vi "fillWithZeros.vi"(9 "string in":string, 11 "width":i32) -> (3 "string out":string)   [LabVIEW 2013, in "Utilities.lvlib"]
uses:
  lib/Utilities.lvlib
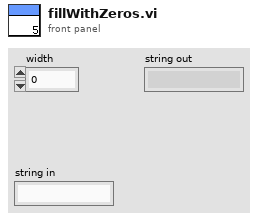
[diagram p1: front panel]
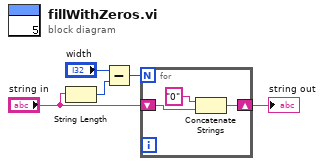
[diagram p0: block diagram]
diagram:
  n1 = String Length(string="string in") -> (length=w2:i32)
  n2 = Subtract(x="width", y=w2) -> (x-y=w4:i32)
  n3 = for {
    N: w4 -> [_]
    shift-right: [w6] -> w5
    shift-left: "string in" -> [w8]
    n4 = Concatenate Strings("0" ("string"), w8) -> (w6:string)
  }
  "string out" <- w5
